vi "Sample_Scanning_Bin_Arrays_V2.vi"(4 "Pixels Per Line":i32=1024, 5 "FPGA Acquisition Clock (MHz)":dbl=200.0, 7 "Scan Rate (Hz)":u32=16) -> (1 "Normalization Array":sgl[](array[numeric]), 2 "Cycles Per Pixel":u32[](array[numeric]))   [LabVIEW 2014]
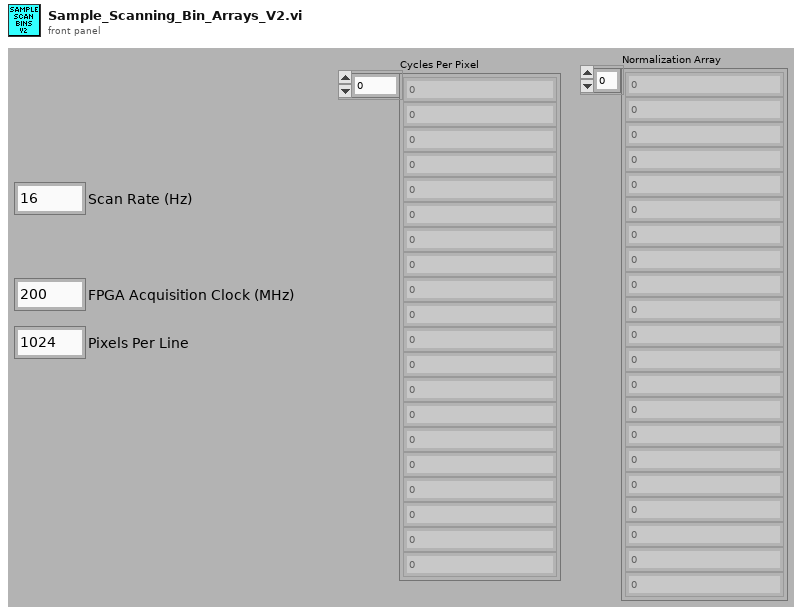
[diagram p1: front panel]
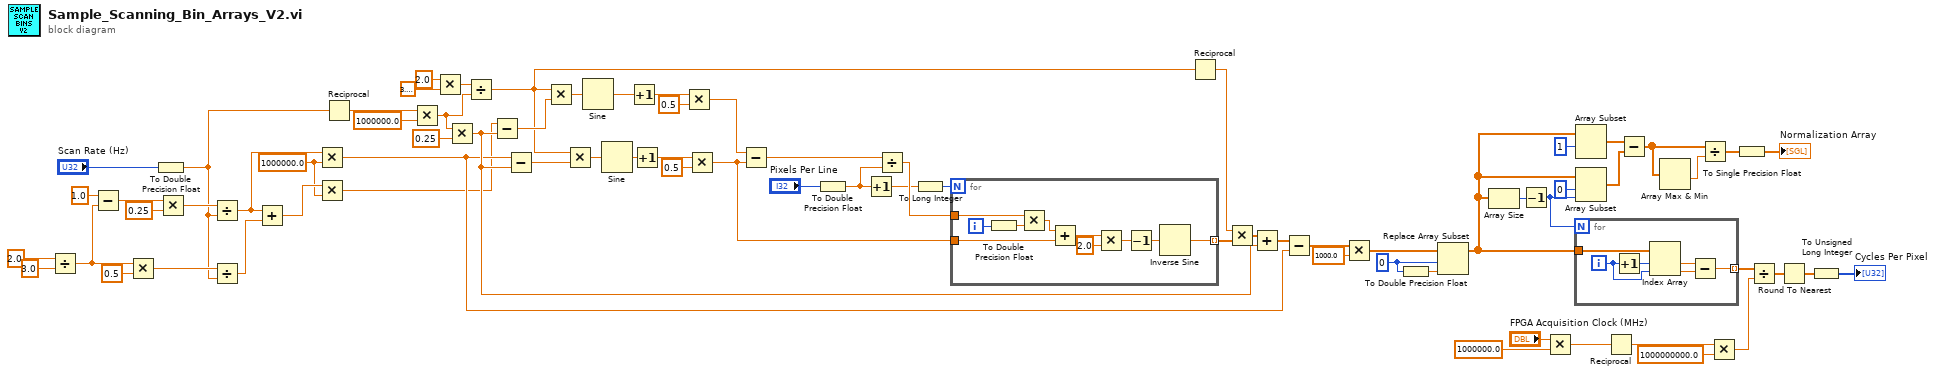
[diagram p0: block diagram]
diagram:
  w31 = 0 ("index")
  w63 = 1000000.0 ("y")
  n1 = Divide(x=2.0, y=3.0) -> (x/y=w72:dbl)
  n2 = Subtract(x=1.0, y=w72) -> (x-y=w71:dbl)
  n3 = Multiply(x=w72, y=0.5) -> (x*y=w74:dbl)
  n4 = To Double Precision Float(number="Scan Rate (Hz)") -> (double precision float=w3:dbl)
  n5 = Multiply(x=w71, y=0.25) -> (x*y=w69:dbl)
  n6 = Divide(x=w69, y=w3) -> (x/y=w53:dbl)
  n7 = Divide(x=w74, y=w3) -> (x/y=w65:dbl)
  n8 = Add(x=w53, y=w65) -> (x+y=w64:dbl)
  n9 = Multiply(x=w53, y=w63) -> (x*y=w25:dbl)
  n10 = Multiply(x=w64, y=w63) -> (x*y=w24:dbl)
  n11 = Reciprocal(x=w3) -> (1/x=w51:dbl)
  n12 = Multiply(x=w51, y=1000000.0) -> (x*y=w50:dbl)
  n13 = Multiply(x=2.0 ("y"), y=3.141592653589793) -> (x*y=w59:dbl)
  n14 = Multiply(x=w50, y=0.25) -> (x*y=w37:dbl)
  n15 = Divide(x=w59, y=w50) -> (x/y=w41:dbl)
  n16 = Subtract(x=w24, y=w37) -> (x-y=w58:dbl)
  n17 = Subtract(x=w25, y=w37) -> (x-y=w45:dbl)
  n18 = Multiply(x=w41, y=w58) -> (x*y=w57:dbl)
  n19 = Multiply(x=w41, y=w45) -> (x*y=w46:dbl)
  n20 = Sine(x=w57) -> (sin(x)=w56:dbl)
  n21 = Sine(x=w46) -> (sin(x)=w47:dbl)
  n22 = Increment(x=w56) -> (x+1=w55:dbl)
  n23 = Increment(x=w47) -> (x+1=w48:dbl)
  n24 = Multiply(x=w55, y=0.5) -> (x*y=w22:dbl)
  n25 = Multiply(x=w48, y=0.5) -> (x*y=w23:dbl)
  n26 = Subtract(x=w22, y=w23) -> (x-y=w44:dbl)
  n27 = To Double Precision Float(number="Pixels Per Line") -> (double precision float=w2:dbl)
  n28 = Increment(x=w2) -> (x+1=w26:dbl)
  n29 = Divide(x=w44, y=w2) -> (x/y=w43:dbl)
  n30 = To Long Integer(number=w26) -> (32bit integer=w42:i32)
  n31 = for {
    N: w42 -> [_]
    tunnel: w23 -> [w84]
    tunnel: w43 -> [w83]
    tunnel: [w76] -> w40 mode=indexing
    i -> [w82]
    n32 = To Double Precision Float(number=w82) -> (double precision float=w81:dbl)
    n33 = Multiply(x=w83, y=w81) -> (x*y=w80:dbl)
    n34 = Add(x=w80, y=w84) -> (x+y=w75:dbl)
    n35 = Multiply(x=w75, y=2.0) -> (x*y=w78:dbl)
    n36 = Decrement(x=w78) -> (x-1=w77:dbl)
    n37 = Inverse Sine(1:w77) -> (0:w76:dbl)
  }
  n38 = Reciprocal(x=w41) -> (1/x=w39:dbl)
  n39 = Multiply(x=w39, y=w40) -> (x*y=w38:dbl[])
  n40 = Add(x=w38, y=w37) -> (x+y=w36:dbl[])
  n41 = Subtract(x=w36, y=w25) -> (x-y=w35:dbl[])
  n42 = Multiply(x=w35, y=1000.0) -> (x*y=w33:dbl[])
  n43 = To Double Precision Float(number=w31) -> (double precision float=w32:dbl)
  n44 = Replace Array Subset(array=w33, new element=w32, index=w31) -> (w13:dbl[])
  n45 = Array Size(array=w13) -> (size(s)=w21:i32)
  n46 = Decrement(x=w21) -> (x-1=w4:i32)
  n47 = Multiply(x="FPGA Acquisition Clock (MHz)", y=1000000.0) -> (x*y=w30:dbl)
  n48 = for {
    N: w4 -> [_]
    tunnel: w13 -> [w90]
    tunnel: [w86] -> w12 mode=indexing
    i -> [w85]
    n49 = Increment(x=w85) -> (x+1=w89:i32)
    n50 = Index Array(array=w90, index #1=w89, index #2=w85) -> (element #1=w88:dbl, element #2=w87:dbl)
    n51 = Subtract(x=w88, y=w87) -> (x-y=w86:dbl)
  }
  n52 = Array Subset(array=w13, index=1) -> (w18:dbl[])  [unwired: 1 in]
  n53 = Array Subset(array=w13, index=0, length=w4) -> (w17:dbl[])
  n54 = Reciprocal(x=w30) -> (1/x=w29:dbl)
  n55 = Subtract(x=w18, y=w17) -> (x-y=w16:dbl[])
  n56 = Array Max & Min(array=w16) -> (min value=w15:dbl)  [unwired: 3 out]
  n57 = Divide(x=w16, y=w15) -> (x/y=w14:dbl[])
  n58 = Multiply(x=w29, y=1000000000.0) -> (x*y=w11:dbl)
  n59 = To Single Precision Float(number=w14) -> (single precision float=→"Normalization Array":sgl[])
  n60 = Divide(x=w12, y=w11) -> (x/y=w9:dbl[])
  n61 = Round To Nearest(number=w9) -> (nearest integer value=w10:dbl[])
  n62 = To Unsigned Long Integer(number=w10) -> (unsigned 32bit integer=→"Cycles Per Pixel":u32[])
